vi "remote command.vi"(4 "User Parameter":variant, 5 "Event Data":cluster{"sender":refnum<k24>, "e":refnum<k24>}, 6 "Control Ref":refnum<k24>, 7 "Event Common Data":T1) -> ()   [LabVIEW 2022 SP3]
uses:
  C:/Software Repos/shared components/SECSGEM/DotNet20EqApp/GemEqApp/SecsPort.dll
  Software Repos/shared components/SECSGEM/DotNet20EqApp/GemEqApp/SecsPort.dll
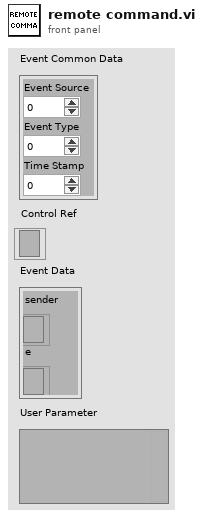
[diagram p1: front panel]
types:
  T1 = cluster{"Event Source":i32, "Event Type":u32, "Time Stamp":u32}
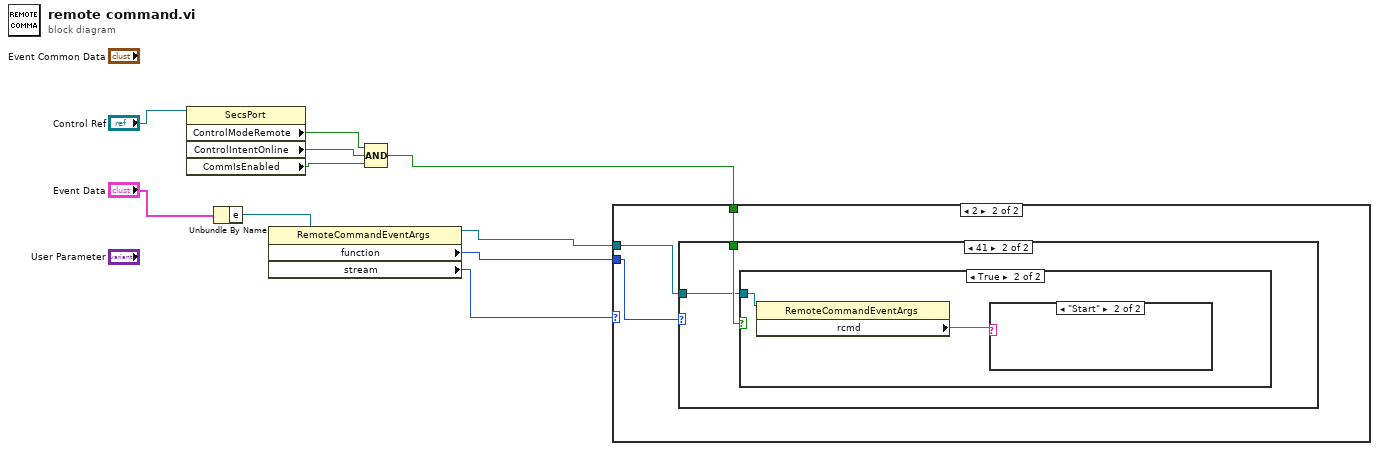
[diagram p0: block diagram]
diagram:
  n1 = property class="SecsPort"(reference="Control Ref") -> ("ControlModeRemote"=w9:bool, "ControlIntentOnline"=w8:bool, "CommIsEnabled"=w7:bool)  [unwired: 1 in, 2 out]
  n2 = Unbundle By Name("Event Data") -> ("e"=w5:refnum<k24>)
  n3 = property class="RemoteCommandEventArgs"(reference=w5) -> (reference out=w1:refnum<k24>, "function"=w3:i32, "stream"=w4:i32)  [unwired: 1 in, 1 out]
  n4 = Compound Arithmetic op=AND(w9, w8, w7) -> (w2:bool)
  n5 = case shown="2" w4 {
    tunnel: w3 -> [_ w13]
    tunnel: w2 -> [_ w12]
    tunnel: w1 -> [_ w11]
    frame 0, Default {
    }
    frame 2 {
      n6 = case shown="41" w13 {
        tunnel: w12 -> [_ w15]
        tunnel: w11 -> [_ w14]
        frame Default {
        }
        frame 41 {
          n7 = case shown="True" w15 {
            tunnel: w14 -> [_ w17]
            frame False {
            }
            frame True {
              n8 = property class="RemoteCommandEventArgs"(reference=w17) -> ("rcmd"=w16:string)  [unwired: 1 in, 2 out]
              n9 = case shown="\"Start\"" w16 {
                frame "False", Default {
                }
                frame "Start" {
                }
              }
            }
          }
        }
      }
    }
  }
